vi "游标显示-开启关闭.vi"(3 "计算参数 in":T1, 5 "reference in":refnum<vi>) -> (0 "计算参数 out":T1, 2 "reference out":refnum<vi>)   [LabVIEW 2013]
panel:
  in  "Array":string[](array[string])=["行程", "油压1"]
  in  "Cursor":T2
  out "Xrange":dbl
  out "Yrange":dbl
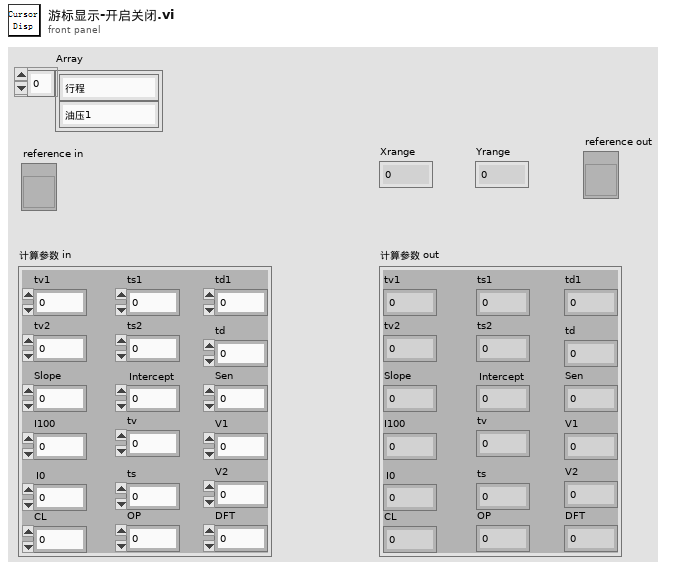
[diagram p1: front panel]
types:
  T1 = cluster{"tv1":dbl, "tv2":dbl, "tv":dbl, "ts1":dbl, "ts2":dbl, "ts":dbl, "td1":dbl, "td":dbl, "Slope":dbl, "Intercept":dbl, "I100":dbl, "I0":dbl, "Sen":dbl, "V1":dbl, "V2":dbl, "CL":dbl, "OP":dbl, "DFT":dbl}
  T2 = cluster{"Name":string, "Color":u32, "Style":u8, "Point Style":u8, "Name Visible":bool, "Allow Drag":bool, "Cursor Mode":u32, "Plot":i32, "Index":i32, "Position":cluster{"X":dbl, "Y":dbl}, "X Scale":u32, "Y Scale":u32, "Watch Plots":i32[], "Watch All Plots":bool, "Plot Area":i32, "Label Offset":cluster{"X":dbl, "Y":dbl}}
  T3 = cluster{"Name":string, "Color":u32, "Style":u8, "Point Style":u8, "Name Visible":bool, "Allow Drag":bool, "Cursor Mode":u32, "Plot":i32, "Index":i32, "Position":cluster{"X":dbl, "Y":dbl}, "X Scale":u32, "Y Scale":u32, "Watch Plots":i32[], "Watch All Plots":bool, "Plot Area":i32, "Label Offset":cluster{"X":dbl, "Y":dbl}}[]
  T4 = typedef "LVCursorListTypeDef.ctl" = cluster{"Name":string, "Color":u32, "Style":u8, "Point Style":u8, "Name Visible":bool, "Allow Drag":bool, "Cursor Mode":u32, "Plot":i32, "Index":i32, "Position":cluster{"X":dbl, "Y":dbl}, "X Scale":u32, "Y Scale":u32, "Watch Plots":i32[], "Watch All Plots":bool, "Plot Area":i32, "Label Offset":cluster{"X":dbl, "Y":dbl}}[]
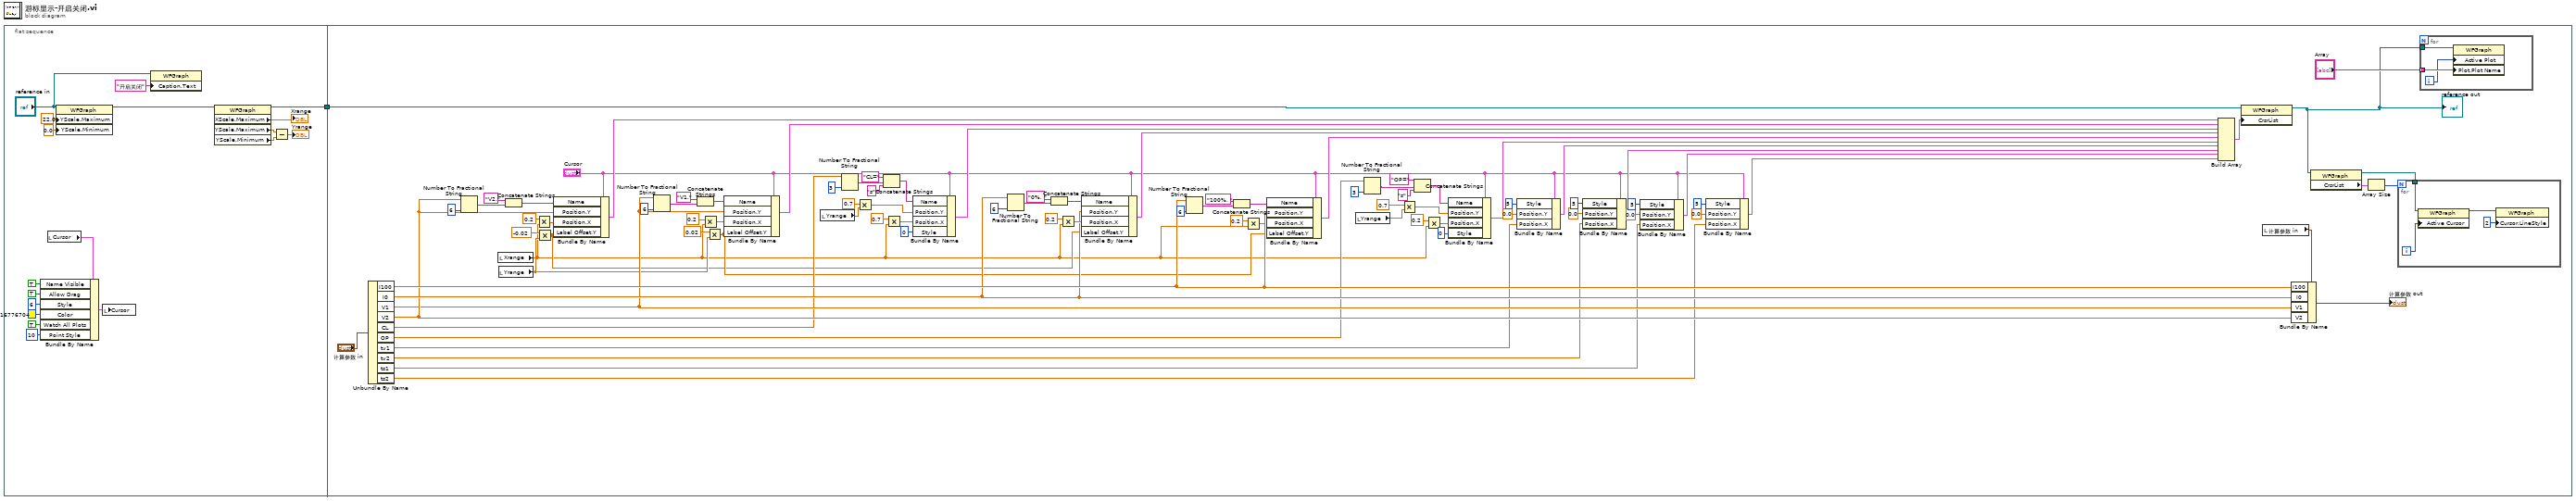
[diagram p0: block diagram]
diagram:
  n1 = flat-sequence {
    tunnel: [w10] -> w1
    tunnel: w1 -> [w58]
    frame #0 {
      n2 = local read "Cursor"() -> (w16:T2)
      n3 = Bundle By Name(cluster=w16, "Name Visible"=TRUE, "Allow Drag"=TRUE, "Style"=u8 6, "Color"=u32 16776704, "Watch All Plots"=TRUE, "Point Style"=u8 10) -> (w15:T2)
      n4 = property on="属性节点" class="WFGraph"(reference="reference in", "YScale.Maximum"=22.0 ("Y标尺.范围:最大值"), "YScale.Minimum"=0.0 ("Y标尺.范围:最小值")) -> (reference out=w2:refnum<vi>)  [unwired: 1 in, 1 out]
      n5 = local write "Cursor"(w15) -> ()
      n6 = property on="Property Node" class="WFGraph"(reference="reference in", "Caption.Text"="开启关闭") -> ()  [unwired: 1 in, 2 out]
      n7 = property class="WFGraph"(reference=w2) -> (reference out=w10:refnum<vi>, "XScale.Maximum"=→"Xrange":dbl, "YScale.Maximum"=w7:dbl, "YScale.Minimum"=w6:dbl)  [unwired: 1 in, 1 out]
      n8 = Subtract(x=w7, y=w6) -> (x-y=→"Yrange":dbl)
    }
    frame #1 {
      n9 = Unbundle By Name("计算参数 in") -> ("I100"=w107:dbl, "I0"=w102:dbl, "V1"=w61:dbl, "V2"=w93:dbl, "CL"=w57:dbl, "OP"=w56:dbl, "tv1"=w45:dbl, "tv2"=w42:dbl, "ts1"=w33:dbl, "ts2"=w32:dbl)
      n10 = Number To Fractional String(number=w93, precision (6)=i16 6 ("宽度(-)")) -> (F-format string=w67:string)  [unwired: 2 in]
      n11 = local read "Xrange"() -> (w22:dbl)
      n12 = local read "Yrange"() -> (w26:dbl)
      n13 = Concatenate Strings("V2," ("光标.游标名"), w67) -> (w92:string)
      n14 = Multiply(x=0.2 ("y"), y=w22) -> (x*y=w94:dbl)
      n15 = Multiply(x=-0.02, y=w26) -> (x*y=w24:dbl)
      n16 = Bundle By Name(cluster="Cursor", "Name"=w92, "Position.Y"=w93, "Position.X"=w94, "Label Offset.Y"=w24) -> (w86:T2)
      n17 = Number To Fractional String(number=w61, precision (6)=i16 6 ("宽度(-)")) -> (F-format string=w64:string)  [unwired: 2 in]
      n18 = Concatenate Strings("V1," ("光标.游标名"), w64) -> (w62:string)
      n19 = Multiply(x=0.2 ("y"), y=w22) -> (x*y=w60:dbl)
      n20 = Multiply(x=0.02, y=w26) -> (x*y=w25:dbl)
      n21 = Bundle By Name(cluster="Cursor", "Name"=w62, "Position.Y"=w61, "Position.X"=w60, "Label Offset.Y"=w25) -> (w59:T2)
      n22 = local read "Yrange"() -> (w101:dbl)
      n23 = Number To Fractional String(number=w57, precision (6)=i16 3 ("宽度(-)")) -> (F-format string=w81:string)  [unwired: 2 in]
      n24 = Multiply(x=0.7 ("y"), y=w101) -> (x*y=w99:dbl)
      n25 = Concatenate Strings("CL=" ("字符串"), w81, "s" ("字符串")) -> (w98:string)
      n26 = Multiply(x=0.7 ("y"), y=w22) -> (x*y=w52:dbl)
      n27 = Bundle By Name(cluster="Cursor", "Name"=w98, "Position.Y"=w99, "Position.X"=w52, "Style"=u8 0) -> (w87:T2)
      n28 = Number To Fractional String(number=w102, precision (6)=i16 6 ("宽度(-)")) -> (F-format string=w70:string)  [unwired: 2 in]
      n29 = Concatenate Strings("0%, " ("光标.游标名"), w70) -> (w96:string)
      n30 = Multiply(x=0.2 ("y"), y=w22) -> (x*y=w104:dbl)
      n31 = Bundle By Name(cluster="Cursor", "Name"=w96, "Position.Y"=w102, "Position.X"=w104, "Label Offset.Y"=w24) -> (w88:T2)
      n32 = Number To Fractional String(number=w107, precision (6)=i16 6 ("宽度(-)")) -> (F-format string=w73:string)  [unwired: 2 in]
      n33 = Concatenate Strings("100%, " ("光标.游标名"), w73) -> (w95:string)
      n34 = Multiply(x=0.2 ("y"), y=w22) -> (x*y=w106:dbl)
      n35 = Bundle By Name(cluster="Cursor", "Name"=w95, "Position.Y"=w107, "Position.X"=w106, "Label Offset.Y"=w25) -> (w89:T2)
      n36 = local read "Yrange"() -> (w110:dbl)
      n37 = Number To Fractional String(number=w56, precision (6)=i16 3 ("宽度(-)")) -> (F-format string=w82:string)  [unwired: 2 in]
      n38 = Multiply(x=0.7 ("y"), y=w110) -> (x*y=w109:dbl)
      n39 = Concatenate Strings("OP=" ("字符串"), w82, "s" ("字符串")) -> (w97:string)
      n40 = Multiply(x=0.2 ("y"), y=w22) -> (x*y=w50:dbl)
      n41 = Bundle By Name(cluster="Cursor", "Name"=w97, "Position.Y"=w109, "Position.X"=w50, "Style"=u8 0) -> (w90:T2)
      n42 = Bundle By Name(cluster="Cursor", "Style"=u8 5, "Position.Y"=0.0, "Position.X"=w45) -> (w37:T2)
      n43 = Bundle By Name(cluster="Cursor", "Style"=u8 5, "Position.Y"=0.0, "Position.X"=w42) -> (w34:T2)
      n44 = Bundle By Name(cluster="Cursor", "Style"=u8 5, "Position.Y"=0.0, "Position.X"=w33) -> (w35:T2)
      n45 = Bundle By Name(cluster="Cursor", "Style"=u8 5, "Position.Y"=0.0, "Position.X"=w32) -> (w36:T2)
      n46 = Build Array(w86, w59, w87, w88, w89, w90, w37, w34, w35, w36) -> (w91:T3)
      n47 = property class="WFGraph"(reference=w58, "CrsrList"=w91) -> (reference out=w20:refnum<vi>)  [unwired: 1 in, 1 out]
      "reference out" <- w20
      n48 = local read "计算参数 in"() -> (w84:T1)
      n49 = Bundle By Name(cluster=w84, "I100"=w107, "I0"=w102, "V1"=w61, "V2"=w93) -> (→"计算参数 out":T1)
      n50 = property class="WFGraph"(reference=w20) -> (reference out=w29:refnum<vi>, "CrsrList"=w31:T4)  [unwired: 1 in, 1 out]
      n51 = Array Size(array=w31) -> (size(s)=w30:i32)
      n52 = for {
        N: w30 -> [_]
        tunnel: w29 -> [w117]
        i -> [w116]
        n53 = property class="WFGraph"(reference=w117, "Active Cursor"=w116) -> (reference out=w115:refnum<vi>)  [unwired: 1 in, 1 out]
        n54 = property class="WFGraph"(reference=w115, "Cursor.LineStyle"=u8 2 ("Cursor.Line Style")) -> ()  [unwired: 1 in, 2 out]
      }
      n55 = for {
        tunnel: "Array" -> [w113] mode=indexing
        tunnel: w20 -> [w112]
        i -> [w111]
        n56 = property class="WFGraph"(reference=w112, "Active Plot"=w111, "Plot.Plot Name"=w113) -> ()  [unwired: 1 in, 2 out]
      }
    }
  }
